vi "to_I16.vi"(8 "error_in":errorcluster, 10 "variable_start_index":i32, 11 "byte_array":u8[](array[numeric])) -> (0 "error_out":errorcluster, 3 "I16":i16)   [LabVIEW 2020]
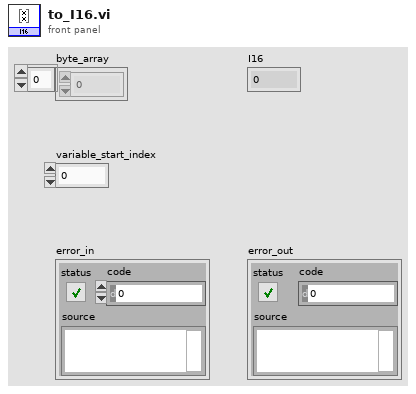
[diagram p1: front panel]
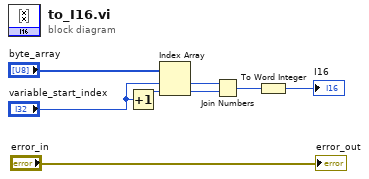
[diagram p0: block diagram]
diagram:
  n1 = Increment(x="variable_start_index") -> (x+1=w5:i32)
  n2 = Index Array(array="byte_array", index #1="variable_start_index", index #2=w5) -> (element #1=w7:u8, element #2=w8:u8)
  n3 = Join Numbers(hi=w7, lo=w8) -> ((hi.lo)=w2:u16)
  n4 = To Word Integer(number=w2) -> (16bit integer=→"I16":i16)
  "error_out" <- "error_in"
